vi "GetProtocolProgress.vi"() -> (2 "percentage":u8(slide) scale=0.0..100.0)   [LabVIEW 2018]
uses:
  <vilib>/addons/_JKI.lib/REST Client/classes/REST Client/REST Client.lvclass
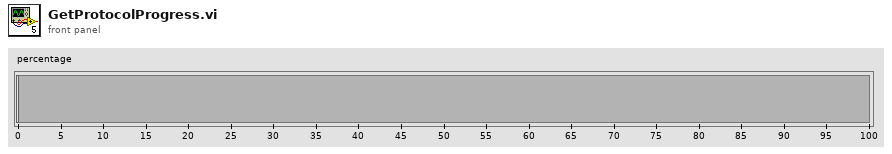
[diagram p1: front panel]
types:
  T1 = cluster{"StartTime":string, "ElapsedTime":string, "RemainingTime":string, "EstimatedTimeOfCompletion":string, "Progress":dbl}
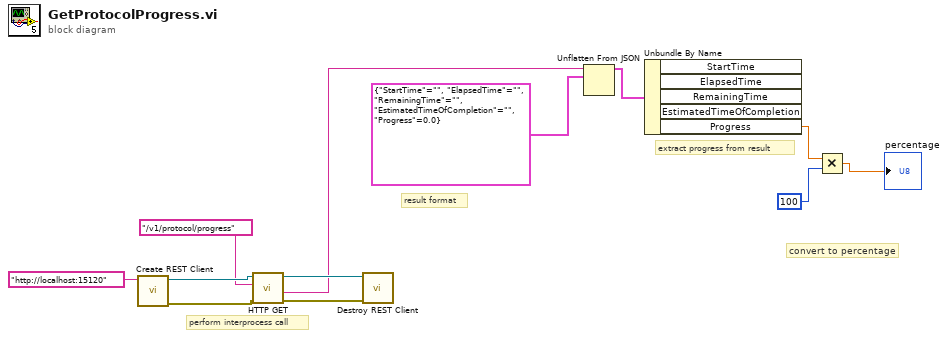
[diagram p0: block diagram]
diagram:
  # "convert to percentage"
  # "extract progress from result"
  # "result format"
  # "perform interprocess call"
  n1 = call <vilib>:"Create REST Client.vi"("Base URL"="http://localhost:15120") -> ("error out"=w10:errorcluster, "REST Client out"=w12:refnum<class "REST Client.lvclass">)  [unwired: 9 in]
  n2 = call-dynamic "HTTP GET.vi"("error in (no error)"=w10, "Path"="/v1/protocol/progress", "REST Client in"=w12) -> ("error out"=w9:errorcluster, "Response body"=w6:string, "REST Client out"=w11:refnum<class "REST Client.lvclass">)  [unwired: 3 in, 3 out]
  n3 = call-dynamic "Destroy REST Client.vi"("error in (no error)"=w9, "REST Client in"=w11) -> ()  [unwired: 9 in, 1 out]
  n4 = Unflatten From JSON(JSON string=w6, type and defaults=T1 {"StartTime"="", "ElapsedTime"="", "RemainingTime"="", "EstimatedTimeOfCompletion"="", "Progress"=0.0}) -> (value=w4:T1)  [unwired: 5 in, 1 out]
  n5 = Unbundle By Name(w4) -> ("Progress"=w3:dbl)  [unwired: 4 out]
  n6 = Multiply(x=w3, y=100) -> (x*y=→"percentage":dbl)
